vi "save_list_fit.vi"(9 "Elements Selected":string[][](table), 10 "list path in":path, 11 "List ROI out":dbl[][](array[numeric])) -> (2 "list path out":path, 3 "list array":string[][](array[string]))   [LabVIEW 2020]
panel:
  out "Number od ROIs":i32
  out "Number of Elements":i32
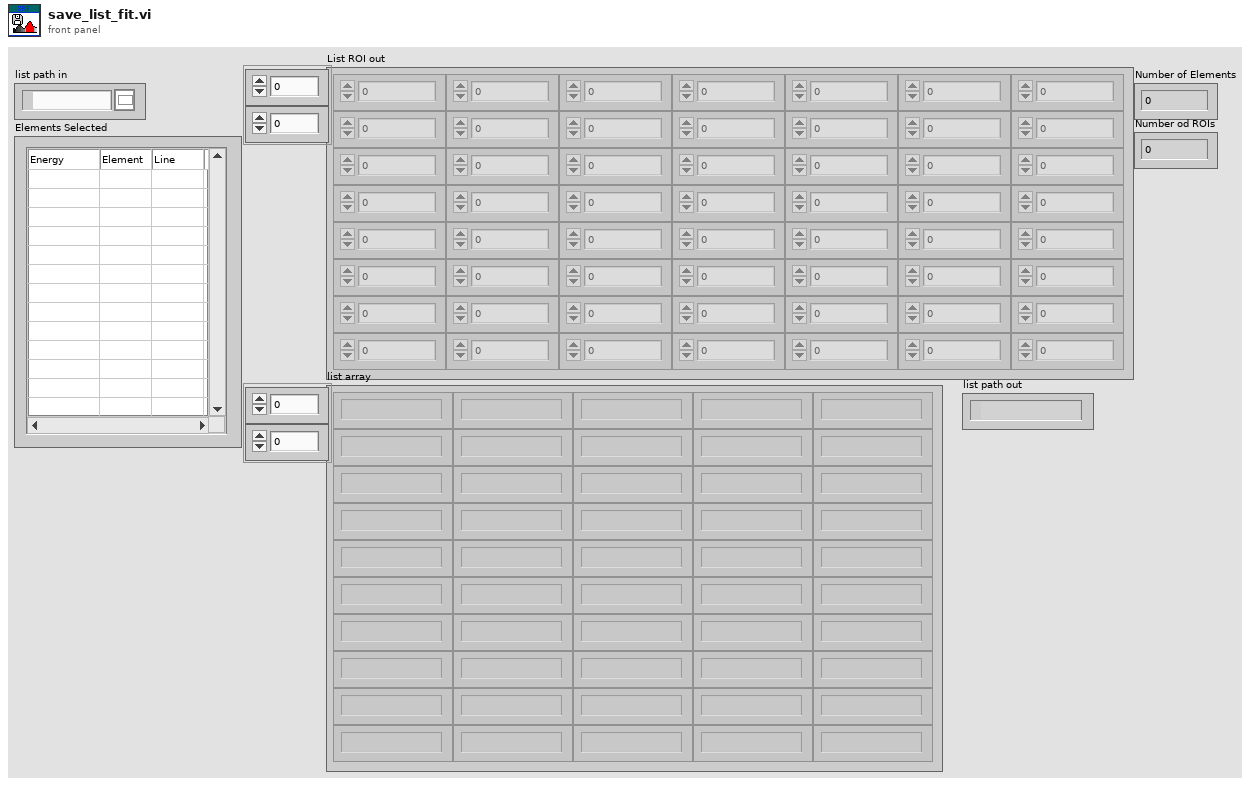
[diagram p1: front panel]
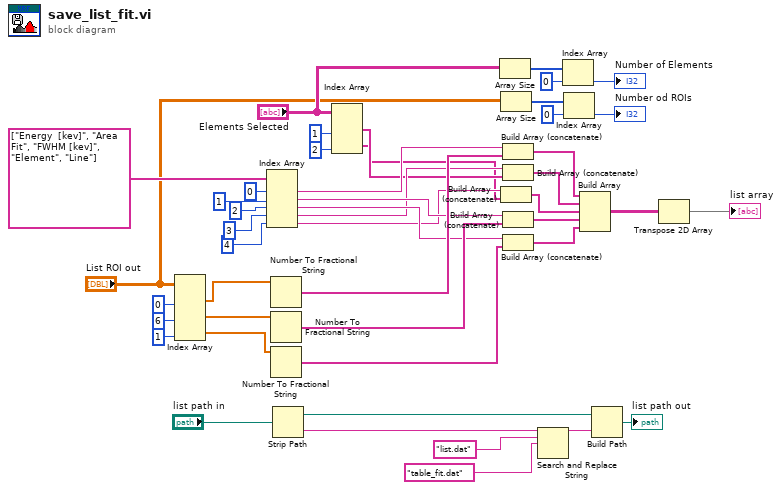
[diagram p0: block diagram]
diagram:
  n1 = Index Array(array="List ROI out", index (col) #1=0 ("disabled index (col)"), index (col) #2=6 ("index (col)"), index (col) #3=1 ("index (col)")) -> (element #1=w43:dbl[], element #2=w42:dbl[], element #3=w41:dbl[])  [unwired: 3 in]
  n2 = Index Array(array=string[] ["Energy  [kev]", "Area Fit", "FWHM [kev]", "Element", "Line"], index #1=0 ("index"), index #2=1 ("index"), index #3=2 ("index"), index #4=3 ("index"), index #5=4 ("index")) -> (element #1=w36:string, element #2=w34:string, element #3=w32:string, element #4=w16:string, element #5=w15:string)
  n3 = Number To Fractional String(number=w43) -> (F-format string=w35:string[])  [unwired: 3 in]
  n4 = Number To Fractional String(number=w42) -> (F-format string=w33:string[])  [unwired: 3 in]
  n5 = Number To Fractional String(number=w41) -> (F-format string=w31:string[])  [unwired: 3 in]
  n6 = Strip Path(path="list path in") -> (stripped path=w21:path, name=w25:string)
  n7 = Index Array(array="Elements Selected", index (col) #1=1 ("disabled index (col)"), index (col) #2=2 ("index (col)")) -> (element #1=w12:string[], element #2=w11:string[])  [unwired: 2 in]
  n8 = Array Size(array="Elements Selected") -> (size(s)=w7:i32[])
  n9 = Array Size(array="List ROI out") -> (size(s)=w5:i32[])
  n10 = Build Array (concatenate)(w15, w11) -> (w10:string[])
  n11 = Build Array (concatenate)(w36, w35) -> (w17:string[])
  n12 = Build Array (concatenate)(w16, w12) -> (w9:string[])
  n13 = Build Array (concatenate)(w34, w33) -> (w30:string[])
  n14 = Build Array (concatenate)(w32, w31) -> (w29:string[])
  n15 = Search and Replace String(input string=w25, search string="list.dat", replace string="table_fit.dat") -> (result string=w22:string)  [unwired: 5 in, 3 out]
  n16 = Index Array(array=w7, index=0) -> (element=→"Number of Elements":i32)
  n17 = Index Array(array=w5, index=0) -> (element=→"Number od ROIs":i32)
  n18 = Build Array(w17, w9, w10, w30, w29) -> (w28:string[][])
  n19 = Build Path(base path=w21, name or relative path=w22) -> (appended path=→"list path out":path)
  n20 = Transpose 2D Array(2D array=w28) -> (transposed array=→"list array":string[][])
